vi "tearDown.vi"(8 "error in (no error)":errorcluster, 11 "reference in":refnum<class "ListImp_Populated.lvclass">) -> (0 "error out":errorcluster, 3 "reference out":refnum<class "ListImp_Populated.lvclass">)   [LabVIEW 2013, in "ListImp_Populated.lvclass"]
doc: "tearDown runs after the test method has completed. Use this method to clean up any operations or references that were opened by setUp or the test method. Unit tests should be independent of other unit tests so this VI should ensure that the next test can run in a 'clean' test environment."
uses:
  ListImp_Populated.lvclass
  ListImp_Populated.lvclass/ListImp_Populated.ctl
  source/LapDog.Collections.Lists/ListImp/ListImp.lvclass
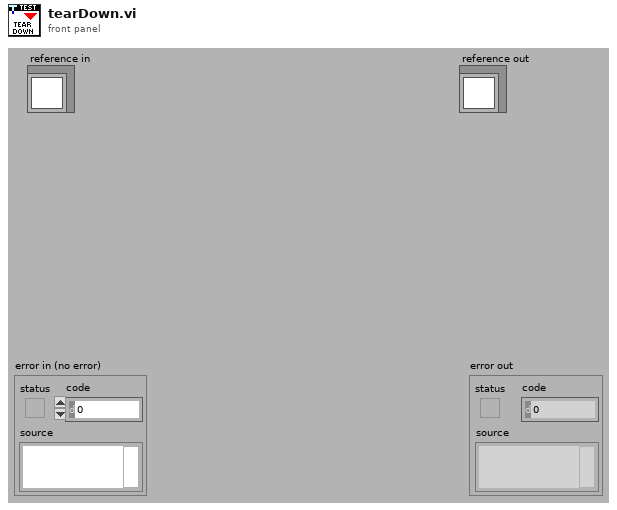
[diagram p1: front panel]
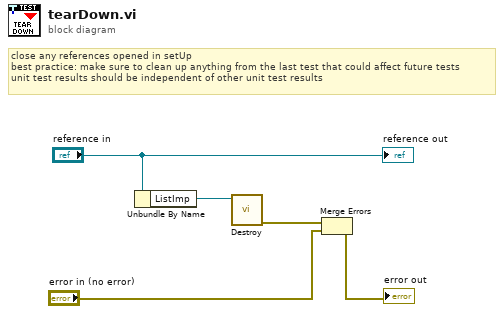
[diagram p0: block diagram]
diagram:
  # "close any references opened in setUp\nbest practice: make sure to clean up anything from the last test that could affect future tests\nunit test results should be independent of other unit test results"
  n1 = Unbundle By Name("reference in") -> ("ListImp"=w2:refnum<class "ListImp.lvclass">)
  n2 = call-dynamic "Destroy.vi"("ListImp in"=w2) -> ("error out"=w1:errorcluster)  [unwired: 10 in]
  n3 = Merge Errors(w1, "error in (no error)") -> (→"error out":errorcluster)
  "reference out" <- "reference in"
